vi "TDT-Enumerate Devices.vi"(11 "error in (no error)":errorcluster, 13 "Acceptable Devices":T2[](array[typedef])=[enum."RX6", enum."RZ5", enum."RZ6"]) -> (8 "Devices":T1[](array[typedef]), 15 "error out":errorcluster)   [LabVIEW 2020]
uses:
  Typedefs/TDT-Device ID.ctl
  Typedefs/TDT-Output source.ctl
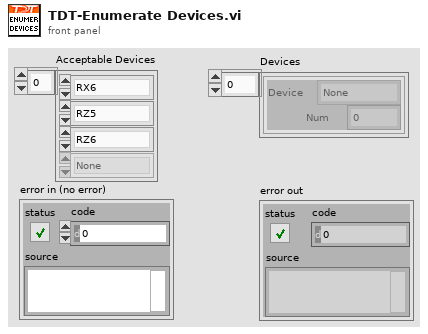
[diagram p1: front panel]
types:
  T1 = typedef "TDT-Output source.ctl" = cluster{"Device":T2, "Num":i32}
  T2 = typedef "TDT-Device ID.ctl" = enum16{"None", "PA5", "RP2", "RL2", "RA16", "RV8", "RX5", "RX6", "RX7", "RX8", "RZ2", "RZ5", "RZ6"}
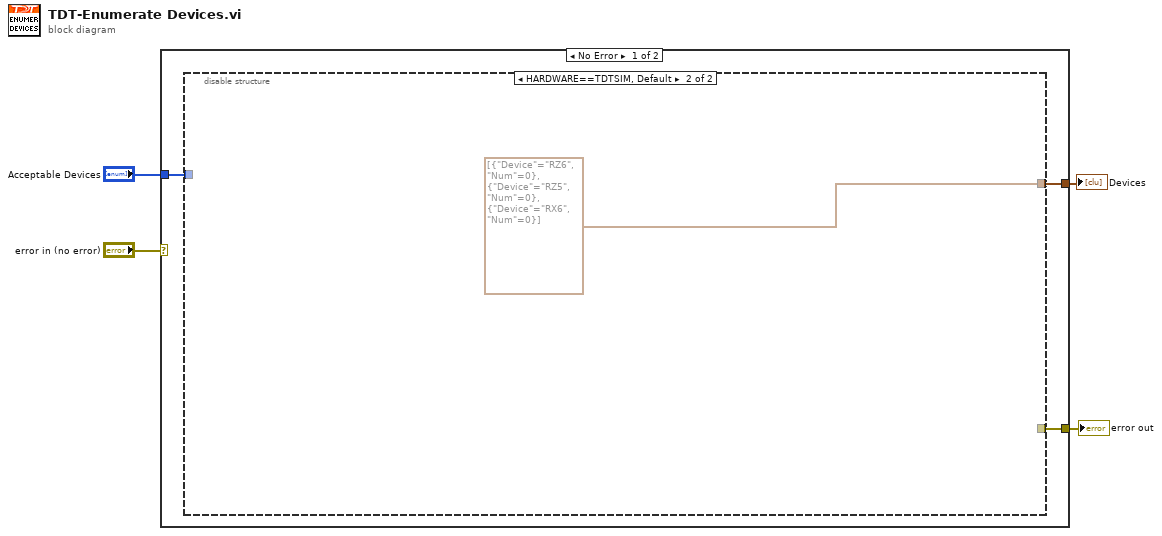
[diagram p0: block diagram]
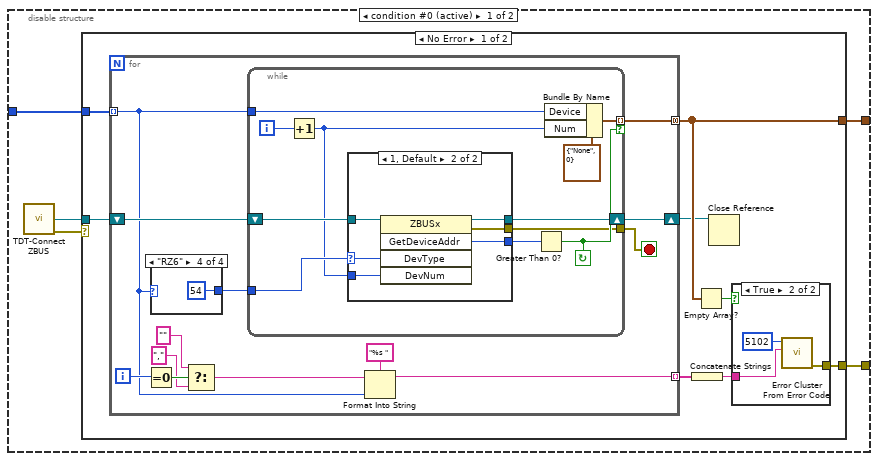
[diagram p2: hidden frame]
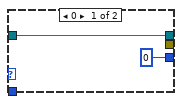
[diagram p4: hidden frame]
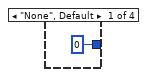
[diagram p5: hidden frame]
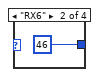
[diagram p6: hidden frame]
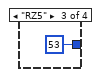
[diagram p7: hidden frame]
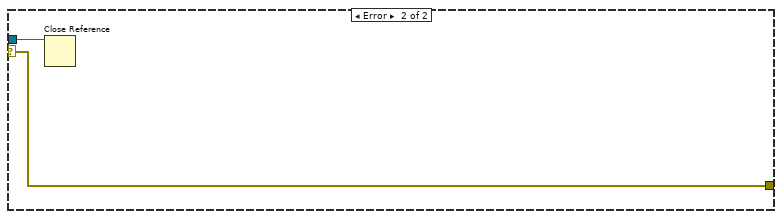
[diagram p8: hidden frame]
diagram:
  n1 = case shown="No Error" "error in (no error)" {
    selector: "error in (no error)" -> [_ w63]
    tunnel: "Acceptable Devices" -> [w7 _]
    tunnel: [w6 _] -> w3
    tunnel: [w5 w63] -> w1
    frame No Error {
      n2 = disable-structure shown="HARDWARE==TDTSIM, Default" {
        disable-tunnel: w7 -> [w12 _]
        disable-tunnel: [w11 T1[] [{"Device"=enum."RZ6", "Num"=0}, {"Device"=enum."RZ5", "Num"=0}, {"Device"=enum."RX6", "Num"=0}]] -> w6
        disable-tunnel: [w10 _] -> w5
        frame condition #0 (active) {
          n3 = call "TDT-Connect ZBUS.vi"() -> ("ZBUSx"=w9:refnum<k7>, "error out"=w8:errorcluster)  [unwired: 14 in]
          n4 = case shown="No Error" w8 {
            selector: w8 -> [_ w61]
            tunnel: w12 -> [w20 _]
            tunnel: [w15 _] -> w11
            tunnel: w9 -> [w19 w60]
            tunnel: [w14 w61] -> w10
            frame No Error {
              n5 = for {
                tunnel: w20 -> [w27] mode=indexing
                tunnel: [w26] -> w15 mode=concatenating
                tunnel: [w33] -> w16 mode=indexing
                shift-right: [w24] -> w13
                shift-left: w19 -> [w36]
                i -> [w32]
                stop <- w25 stop-if-true
                n6 = Equal To 0?(x=w32) -> (x = 0?=w31:bool)
                n7 = case shown="\"RZ6\"" w27 {
                  tunnel: [0 ("DevType") 46 ("DevType") 53 ("DevType") 54 ("DevType")] -> w35
                  frame "None", Default {
                  }
                  frame "RX6" {
                  }
                  frame "RZ5" {
                  }
                  frame "RZ6" {
                  }
                }
                n8 = Select(t="", s=w31, f=",") -> (s? t:f=w29:string)
                n9 = while {
                  tunnel: w35 -> [w46]
                  tunnel: w27 -> [w44]
                  tunnel: [w43] -> w26 mode=indexing if=w42
                  tunnel: [w40] -> w25
                  shift-right: [w37] -> w24
                  shift-left: w36 -> [w47]
                  i -> [w41]
                  stop <- w42 continue-if-true
                  n10 = Increment(x=w41) -> (x+1=w38:i32)
                  n11 = case shown="1, Default" w46 {
                    selector: w46 -> [_ w54]
                    tunnel: w47 -> [w48 w55]
                    tunnel: [_ w53] -> w40
                    tunnel: w38 -> [_ w52]
                    tunnel: [0 ("DevNum") w51] -> w39
                    tunnel: [w48 w50] -> w37
                    frame 0 {
                    }
                    frame 1, Default {
                      n12 = invoke class="ZBUSx" method="GetDeviceAddr"(reference=w55, "DevType"=w54, "DevNum"=w52) -> (reference out=w50:refnum<k7>, error out=w53:errorcluster, "GetDeviceAddr"=w51:i32)  [unwired: 2 in, 2 out]
                    }
                  }
                  n13 = Greater Than 0?(x=w39) -> (x > 0?=w42:bool)
                  n14 = Bundle By Name(cluster=T1 {"Device"=enum."None", "Num"=0} ("Output"), "Device"=w44, "Num"=w38) -> (w43:T1)
                }
                n15 = Format Into String(format string="%s ", initial string=w29, w27) -> (resulting string=w33:string)  [unwired: 1 in, 1 out]
              }
              n16 = Concatenate Strings(w16) -> (w18:string)
              n17 = Empty Array?(array=w15) -> (empty?=w17:bool)
              n18 = Close Reference(reference=w13) -> ()  [unwired: 1 in, 1 out]
              n19 = case shown="True" w17 {
                tunnel: [_ w23] -> w14
                tunnel: w18 -> [_ w21]
                frame False {
                }
                frame True {
                  n20 = call <vilib>:"Error Cluster From Error Code.vi"("error message (\"\")"=w21, "error code (0)"=5102) -> ("error out"=w23:errorcluster)  [unwired: 7 in]
                }
              }
            }
            frame Error {
              n21 = Close Reference(reference=w60) -> ()  [unwired: 1 in, 1 out]
            }
          }
        }
        frame condition #1 {
        }
      }
    }
    frame Error {
    }
  }
  "error out" <- w1
  "Devices" <- w3
